vi "Config_DEACTIVATED.vi"(7 "ACTIVE":bool, 8 "error in (no error)":errorcluster, 9 "PORT":dbl=1.0 min=1.0 max=4.0 step=1.0, 10 "IOLINK MASTER NR":dbl=1.0 min=1.0 max=10.0 step=1.0, 11 "IP":string="192.168.23.100") -> (0 "error out":errorcluster)   [LabVIEW 2022 SP3]
uses:
  <vilib>/NI/Advanced HTTP Client/POST (Buffer).vi
  <vilib>/NI/Advanced HTTP Client/Session.lvclass
panel:
  # "PORT initializing"
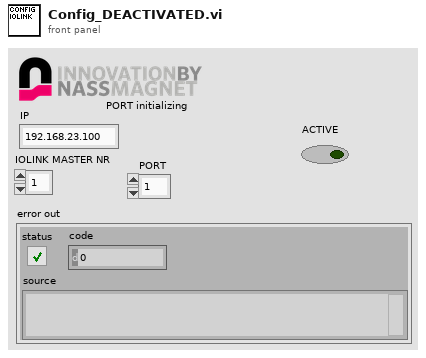
[diagram p1: front panel]
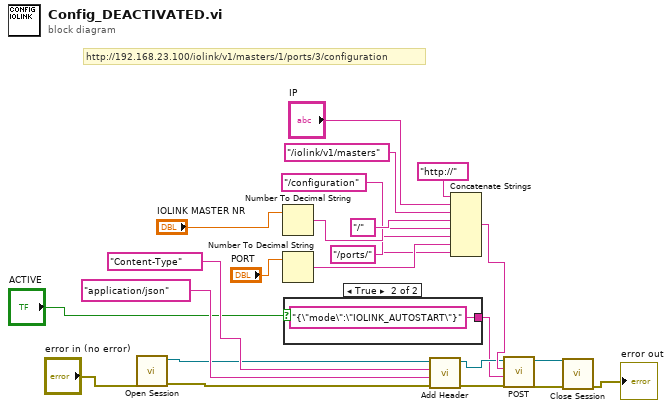
[diagram p0: block diagram]
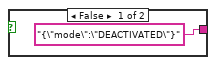
[diagram p2: hidden frame]
diagram:
  # "http://192.168.23.100/iolink/v1/masters/1/ports/3/configuration"
  n1 = call <vilib>:"Open Session.vi"("error in"="error in (no error)") -> ("error out"=w7:errorcluster, "session"=w6:refnum<class "Session.lvclass">)  [unwired: 9 in]
  n2 = Number To Decimal String(number="IOLINK MASTER NR") -> (decimal integer string=w21:string)  [unwired: 1 in]
  n3 = Number To Decimal String(number="PORT") -> (decimal integer string=w17:string)  [unwired: 1 in]
  n4 = case shown="True" "ACTIVE" {
    tunnel: ["{\"mode\":\"DEACTIVATED\"}" ("buffer") "{\"mode\":\"IOLINK_AUTOSTART\"}" ("buffer")] -> w1
    frame False {
    }
    frame True {
    }
  }
  n5 = call <vilib>:"Add Header.vi"("error in"=w7, "value"="application/json" ("buffer"), "header"="Content-Type", "session in"=w6) -> ("error out"=w4:errorcluster, "session out"=w3:refnum<class "Session.lvclass">)  [unwired: 6 in]
  n6 = Concatenate Strings("http://", "IP", "/iolink/v1/masters" ("string"), "/", w21, "/ports/", w17, "/configuration") -> (w14:string)
  n7 = call-poly <vilib>:"POST.vi"("error in"=w4, "buffer"=w1, "url"=w14, "session in"=w3) -> ("error out"=w8:errorcluster, "session out"=w5:refnum<class "Session.lvclass">)  [unwired: 3 in, 3 out]
  n8 = call <vilib>:"Close Session.vi"("error in"=w8, "session"=w5) -> ("error out"=→"error out":errorcluster)  [unwired: 9 in]
